vi "elapsedTime.vi"(8 "error in (no error)":errorcluster, 11 "Model in":refnum<class "Model.lvclass">) -> (0 "error out":errorcluster, 2 "elapsed Time":dbl, 3 "Model out":refnum<class "Model.lvclass">)   [LabVIEW 2016, in "Model.lvclass"]
uses:
  Model.lvclass
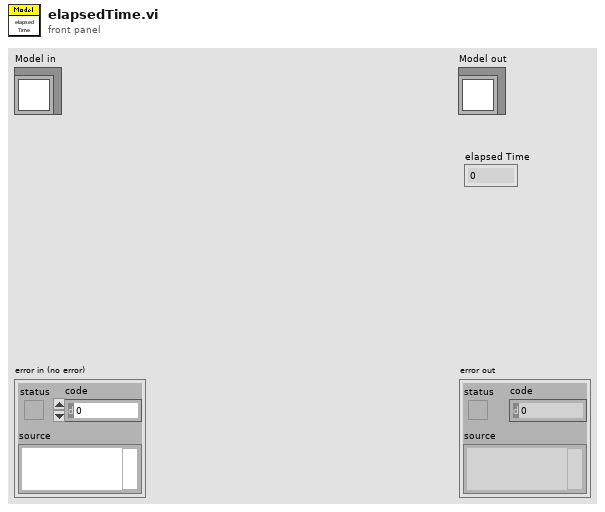
[diagram p1: front panel]
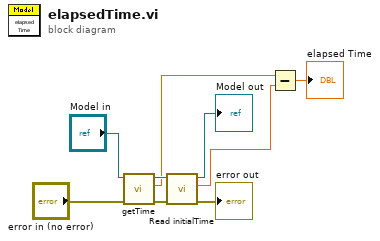
[diagram p0: block diagram]
diagram:
  n1 = call-dynamic "getTime.vi"("error in (no error)"="error in (no error)", "Model in"="Model in") -> ("error out"=w7:errorcluster, "Current Time"=w2:dbl, "Model out"=w6:refnum<class "Model.lvclass">)  [unwired: 7 in]
  n2 = call-dynamic "Read initialTime.vi"("error in (no error)"=w7, "Model in"=w6) -> ("error out"=→"error out":errorcluster, "initial Time"=w1:dbl, "Model out"=→"Model out":refnum<class "Model.lvclass">)  [unwired: 7 in]
  n3 = Subtract(x=w2, y=w1) -> (x-y=→"elapsed Time":dbl)
